vi "to_json.vi"(8 "error in":errorcluster, 11 "s3 in":refnum<class "s3.lvclass">) -> (0 "error out":errorcluster, 2 "json":string, 3 "s3 out":refnum<class "s3.lvclass">)   [LabVIEW 2020, in "datasources.lvlib" / "s3.lvclass"]
uses:
  s3.lvclass
  C:/code/labview-client/lv_src/Nominal Client/datasources/source/source.lvclass
  source/source.lvclass/source.ctl
  b507f1fd-3569-41e4-9012-7a89e1841568.vi
  source/path.get.vi
  <vilib>/JDP Science/JSONtext/Variant to JSON Text.vi
  <vilib>/JDP Science/JSONtext/LVClass Serializer/JSONtext LVClass Serializer.lvclass
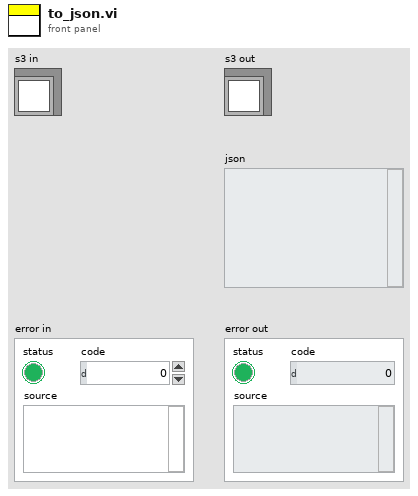
[diagram p1: front panel]
types:
  T1 = cluster{"type":string, "s3":cluster{"path":string}}
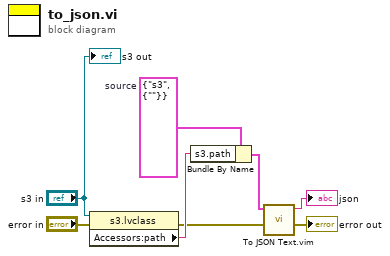
[diagram p0: block diagram]
diagram:
  w7 = T1 {"type"="s3", "s3"={"path"=""}}  # source
  n1 = property class="s3.lvclass"(reference="s3 in", error in="error in") -> (error out=w1:errorcluster, "Accessors:path"=w8:string)  [unwired: 1 out]
  n2 = Bundle By Name(cluster=w7, "s3.path"=w8) -> (w6:T1)
  n3 = call "To JSON Text.vim"("error in (no error)"=w1, "Anything"=w6) -> ("error out"=→"error out":errorcluster, "<JSON>"=→"json":string)  [unwired: 8 in]
  "s3 out" <- "s3 in"
